vi "OpenG Remove Duplicates from 1 D Array Template.vi"() -> ()   [LabVIEW 2018]
panel:
  out "indices of removed elements":i32[](array[numeric])
  out "Output Array":variant[](array[variant])
  in  "Input Array":variant[](array[variant])
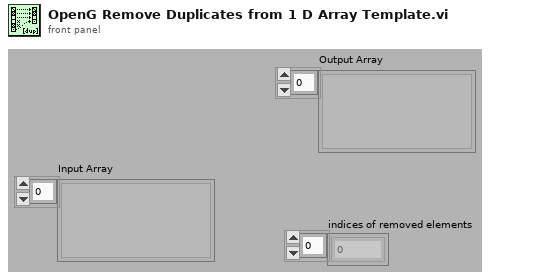
[diagram p1: front panel]
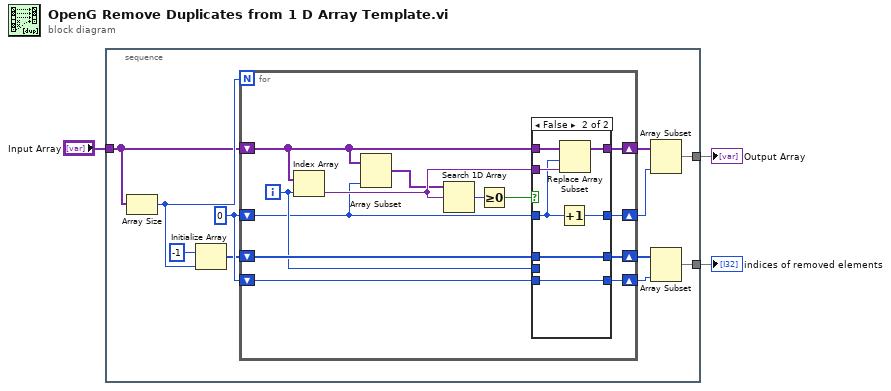
[diagram p0: block diagram]
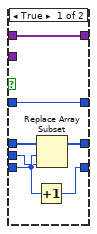
[diagram p2: hidden frame]
diagram:
  n1 = stacked-sequence {
    tunnel: "Input Array" -> [w6]
    tunnel: [w5] -> w2
    tunnel: [w4] -> w1
    frame #0 {
      w9 = 0
      n2 = Array Size(array=w6) -> (size(s)=w13:i32)
      n3 = Initialize Array(-1, w13) -> (w8:i32[])
      n4 = for {
        N: w13 -> [_]
        shift-right: [w27] -> w10
        shift-left: w6 -> [w19]
        shift-right: [w23] -> w12
        shift-left: w8 -> [w24]
        shift-right: [w22] -> w14
        shift-left: w9 -> [w15]
        shift-right: [w25] -> w11
        shift-left: w9 -> [w26]
        i -> [w18]
        n5 = Index Array(array=w19, index=w18) -> (element=w21:variant)
        n6 = Array Subset(array=w19, length=w15) -> (w16:variant[])  [unwired: 1 in]
        n7 = Search 1D Array(1D array=w16, element=w21) -> (index of element=w17:i32)  [unwired: 1 out]
        n8 = Greater Or Equal To 0?(x=w17) -> (x >= 0?=w20:bool)
        n9 = case shown="False" w20 {
          tunnel: w19 -> [w34 w41]
          tunnel: w15 -> [w28 w36]
          tunnel: w21 -> [_ w40]
          tunnel: [w34 w39] -> w27
          tunnel: w26 -> [w33 w38]
          tunnel: [w32 w38] -> w25
          tunnel: w24 -> [w31 w37]
          tunnel: w18 -> [w30 _]
          tunnel: [w29 w37] -> w23
          tunnel: [w28 w35] -> w22
          frame True {
            n10 = Increment(x=w33) -> (x+1=w32:i32)
            n11 = Replace Array Subset(array=w31, new element=w30, index=w33) -> (w29:i32[])
          }
          frame False {
            n12 = Increment(x=w36) -> (x+1=w35:i32)
            n13 = Replace Array Subset(array=w41, new element=w40, index=w36) -> (w39:variant[])
          }
        }
      }
      n14 = Array Subset(array=w10, length=w14) -> (w5:variant[])  [unwired: 1 in]
      n15 = Array Subset(array=w12, length=w11) -> (w4:i32[])  [unwired: 1 in]
    }
  }
  "Output Array" <- w2
  "indices of removed elements" <- w1
